vi "Actor Core.vi"(8 "error in":errorcluster, 11 "Parent in":refnum<class "Message_Distributor_Class.lvclass">) -> (0 "error out":errorcluster, 3 "Actor out":refnum<class "Actor.lvclass">)   [LabVIEW 2023, in "Actor_Message_Distributor.lvlib" / "Message_Distributor_Class.lvclass"]
doc: "(<B>Filename</B>: Actor Framework.lvlib:Actor.lvclass:Actor Core.vi)\n\nReceives messages to the actor, reacts to them, and initiates any error handling that may shut the actor down.\n\nDescendant classes may override this VI to append parallel tasks for the actor to complete while it handles messages. Overrides use the Call Parent Class Method node."
uses:
  Message_Distributor_Class.lvclass
  <vilib>/ActorFramework/Actor/Actor.lvclass
  Message_Distributor_Class.lvclass/Message_Distributor_Class.ctl
  Abstraction_Interface_Class/Abstraction_Interface_Class.lvclass
panel:
  out "Actor_Name":string
  in  "Console":string
  # "DISTRIBUTOR"
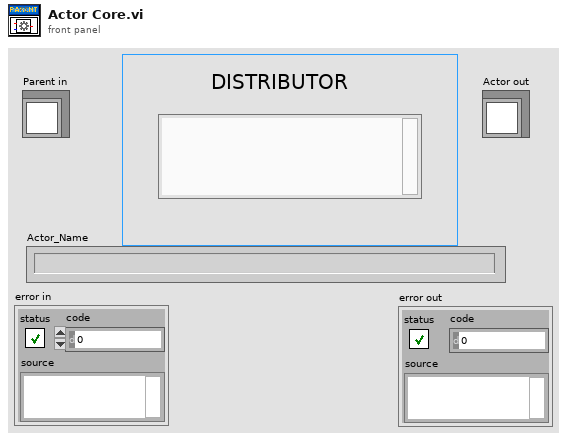
[diagram p1: front panel]
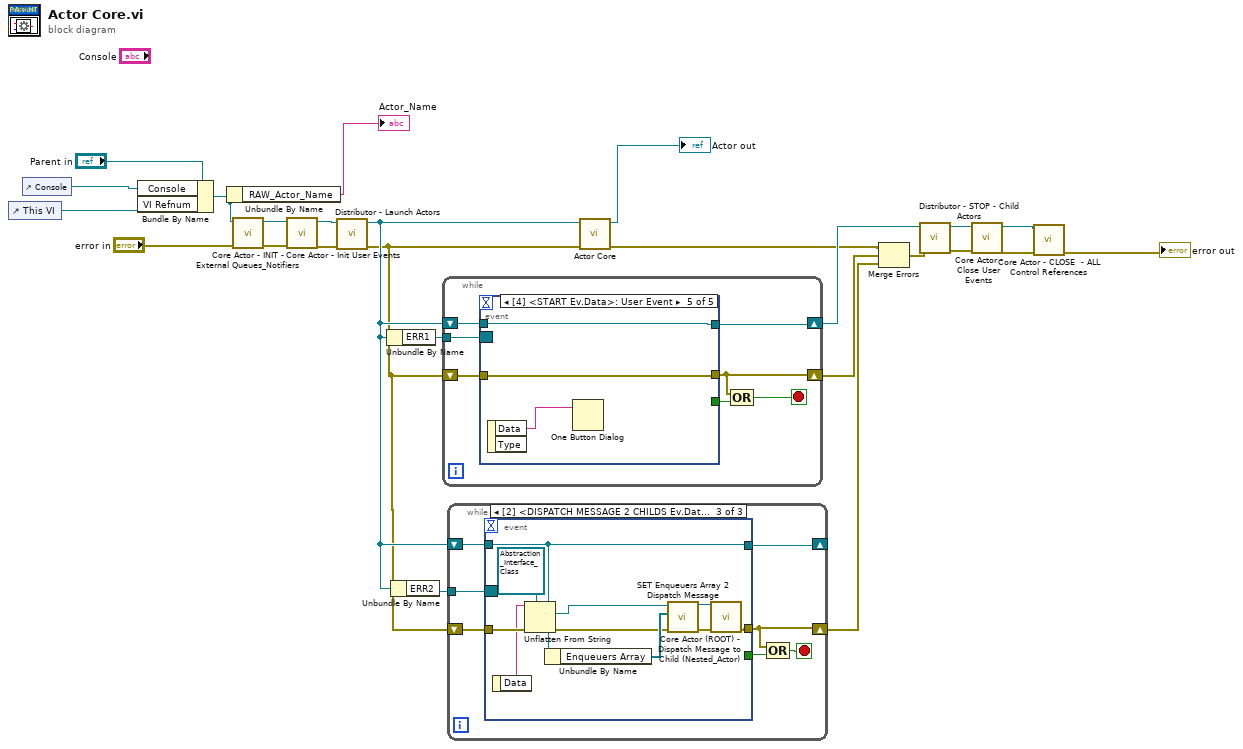
[diagram p0: block diagram]
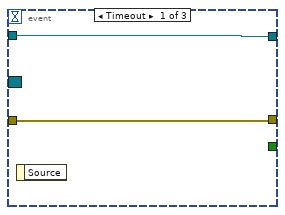
[diagram p2: hidden frame]
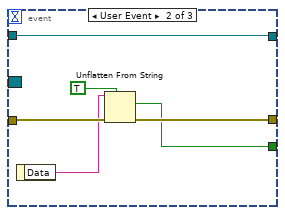
[diagram p3: hidden frame]
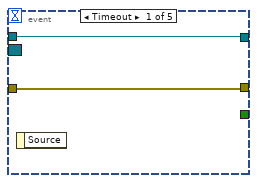
[diagram p4: hidden frame]
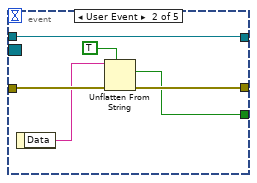
[diagram p5: hidden frame]
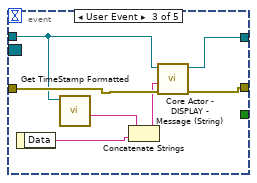
[diagram p6: hidden frame]
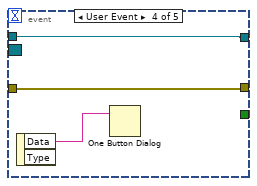
[diagram p7: hidden frame]
diagram:
  n1 = control-ref of="This VI"() -> (w15:refnum<vi>)
  n2 = control-ref of="Console"() -> (w16:refnum<vi>)
  n3 = Bundle By Name(cluster="Parent in", "Console"=w16, "VI Refnum"=w15) -> (w2:refnum<class "Message_Distributor_Class.lvclass">)
  n4 = Unbundle By Name(w2) -> ("RAW_Actor_Name"=→"Actor_Name":string)
  n5 = call-dynamic "Core Actor - INIT - External Queues_Notifiers.vi"("error in (no error)"="error in", "Parent_Class in"=w2) -> ("error out"=w20:errorcluster, "Parent_Class out"=w18:refnum<class "Message_Distributor_Class.lvclass">)  [unwired: 8 in]
  n6 = call-dynamic "Core Actor - Init User Events.vi"("error in (no error)"=w20, "Parent_Class in"=w18) -> ("error out"=w24:errorcluster, "Parent_Class out"=w23:refnum<class "Message_Distributor_Class.lvclass">)  [unwired: 8 in]
  n7 = call "Distributor - Launch Actors.vi"("error in (no error)"=w24, "Parent_Class in"=w23) -> ("error out"=w4:errorcluster, "Parent_Class out"=w5:refnum<class "Message_Distributor_Class.lvclass">)  [unwired: 8 in]
  n8 = Unbundle By Name(w5) -> ("ERR1"=w7:refnum<event-registration>)
  n9 = Unbundle By Name(w5) -> ("ERR2"=w6:refnum<event-registration>)
  n10 = while {
    shift-right: [w28] -> w8
    shift-left: w4 -> [w30]
    shift-right: [w31] -> w11
    shift-left: w5 -> [w32]
    tunnel: w7 -> [w29]
    stop <- w26 stop-if-true
    n11 = event shown="[4] <START Ev.Data>: User Event" {
      selector: w29 -> [_ _ _ _ _]
      dyn-events: _ -> [_ _ _ _ _]
      timeout: _ -> [_ _ _ _ _]
      tunnel: w32 -> [w34 w35 w43 w48 w51]
      tunnel: [w34 w35 w46 w48 w51] -> w31
      tunnel: w30 -> [w33 w40 w45 w50 w53]
      tunnel: [w33 w37 w47 w50 w53] -> w28
      tunnel: [_ w36 _ _ _] -> w27
      event Timeout {
        n12 = event-data() -> ()  [unwired: 1 in, 1 out]
      }
      event User Event {
        n13 = event-data() -> ("Data"=w39:string)  [unwired: 1 in]
        n14 = Unflatten From String(type=TRUE, binary string=w39, error in (no error)=w40) -> (value=w36:bool, error out=w37:errorcluster)  [unwired: 2 in, 1 out]
      }
      event User Event {
        n15 = event-data() -> ("Data"=w44:string)  [unwired: 1 in]
        n16 = call-dynamic "Get TimeStamp Formatted.vi"("Parent in"=w43) -> ("TimeStamp Formatted"=w42:string)  [unwired: 8 in, 2 out]
        n17 = Concatenate Strings(w42, w44) -> (w41:string)
        n18 = call-dynamic "Core Actor - DISPLAY - Message (String).vi"("error in (no error)"=w45, "Value"=w41, "Parent_Class in"=w43) -> ("error out"=w47:errorcluster, "Parent_Class out"=w46:refnum<class "Message_Distributor_Class.lvclass">)  [unwired: 7 in]
      }
      event User Event {
        n19 = event-data() -> ("Data"=w49:string)  [unwired: 1 in, 1 out]
        n20 = One Button Dialog(message=w49) -> ()  [unwired: 1 in, 1 out]
      }
      event User Event {
        n21 = event-data() -> ("Data"=w52:string)  [unwired: 1 in, 1 out]
        n22 = One Button Dialog(message=w52) -> ()  [unwired: 1 in, 1 out]
      }
    }
    n23 = Compound Arithmetic op=OR(w28, w27) -> (w26:bool)
  }
  n24 = while {
    shift-right: [w56] -> w3
    shift-left: w4 -> [w58]
    shift-right: [w59] -> _
    shift-left: w5 -> [w60]
    tunnel: w6 -> [w57]
    stop <- w54 stop-if-true
    n25 = event shown="[2] <DISPATCH MESSAGE 2 CHILDS Ev.Data>: User Event" {
      selector: w57 -> [_ _ _]
      dyn-events: _ -> [_ _ _]
      timeout: _ -> [_ _ _]
      tunnel: w60 -> [w62 w63 w72]
      tunnel: [w62 w63 w72] -> w59
      tunnel: w58 -> [w61 w68 w78]
      tunnel: [w61 w65 w75] -> w56
      tunnel: [_ w64 _] -> w55
      event Timeout {
        n26 = event-data() -> ()  [unwired: 1 in, 1 out]
      }
      event User Event {
        n27 = event-data() -> ("Data"=w67:string)  [unwired: 1 in]
        n28 = Unflatten From String(type=TRUE, binary string=w67, error in (no error)=w68) -> (value=w64:bool, error out=w65:errorcluster)  [unwired: 2 in, 1 out]
      }
      event User Event {
        n29 = event-data() -> ("Data"=w77:string)  [unwired: 1 in]
        n30 = Unflatten From String(type=refnum<class "Abstraction_Interface_Class.lvclass"> refnum ("Actor_Interface.lvlib:Interface_Class.lvclass"), binary string=w77, error in (no error)=w78) -> (value=w74:refnum<class "Abstraction_Interface_Class.lvclass">, error out=w70:errorcluster)  [unwired: 2 in, 1 out]
        n31 = Unbundle By Name(w72) -> ("Enqueuers Array"=w71:refnum<class "Message Enqueuer.lvclass">[])
        n32 = call-dynamic "SET Enqueuers Array 2 Dispatch Message.vi"("error in (no error)"=w70, "Enqueuers Array"=w71, "Interface_Class in"=w74) -> ("error out"=w69:errorcluster, "Interface_Class out"=w73:refnum<class "Abstraction_Interface_Class.lvclass">)  [unwired: 7 in]
        n33 = call-dynamic "Core Actor (ROOT) - Dispatch Message to Child (Nested_Actor).vi"("error in (no error)"=w69, "Interface_Class in"=w73) -> ("error out"=w75:errorcluster)  [unwired: 8 in, 1 out]
      }
    }
    n34 = Compound Arithmetic op=OR(w56, w55) -> (w54:bool)
  }
  n35 = call-parent "Actor Core.vi"("error in"=w4, "Actor in"=w5) -> ("error out"=w9:errorcluster, "Actor out"=→"Actor out":refnum<class "Actor.lvclass">)  [unwired: 8 in]
  n36 = Merge Errors(w9, w8, w3) -> (w10:errorcluster)
  n37 = call "Distributor - STOP - Child Actors.vi"("error in (no error)"=w10, "Parent_Class in"=w11) -> ("error out"=w22:errorcluster, "Parent_Class out"=w21:refnum<class "Message_Distributor_Class.lvclass">)  [unwired: 8 in]
  n38 = call-dynamic "Core Actor - Close User Events.vi"("error in (no error)"=w22, "Parent_Class in"=w21) -> ("error out"=w14:errorcluster, "Parent_Class out"=w13:refnum<class "Message_Distributor_Class.lvclass">)  [unwired: 8 in]
  n39 = call-dynamic "Core Actor - CLOSE  - ALL Control References.vi"("error in (no error)"=w14, "Parent_Class in"=w13) -> ("error out"=→"error out":errorcluster)  [unwired: 8 in, 1 out]
